vi "ADIS16470 Loop.vi"(8 "error in":errorcluster, 9 "Calibration Time":T5, 11 "ADIS16470DevRef":T7={"DevStatus"={"status"=FALSE, "code"=0, "source"=""}, "Hardware Config"={"SPI Clock Rate (Hz)"=1000000.0, "IMU SPI Mode (3)"=enum."Mode 3 (Clk Idle High,Sample on Trailing)", "IMU Reset Pin"=enum."SPI Port CS2", "IMU SPI Bus"=enum."SPI On-Board, CS0", "IMU Data Ready Pin"=enum."SPI Port CS1", "Stall Config"={"Pow2BytesPerRead"=255, "StallTicks"=640, "CsToSclkTicks"=5}}, "Calibration Complete"=refnum, "Status FIFO"=refnum, "Last Value Reference"=refnum, "Sychronous Process VI"=refnum, "Cmd FIFO"=refnum, "Source"={"DevStatus"={"status"=FALSE, "code"=0, "source"=""}, "AnalogTriggerMode?"=FALSE, "DigitalMode"={"DIO Channel"=enum."Disabled"}, "AnalogTriggerMode"={"AnalogTriggerIndex"=enum."Trig 0", "OutputType"=enum."InWindow"}}, "Data FIFO"=refnum, "Calibration Time"=enum."1s"}) -> ()   [LabVIEW 2019]
uses:
  Typedef/ADIS16470 Device Reference.ctl
  Typedef/ADIS16470 Hardware Configuration.ctl
  <vilib>/Rock Robotics/WPI/SPI/WPI_SPIMode.ctl
  <vilib>/Rock Robotics/SystemInterfaces/DIO/FPGA_DIOChannel.ctl
  <vilib>/Rock Robotics/SystemInterfaces/spilib/spi_bus.ctl
  Typedef/ADIS16470 Status.ctl
  Typedef/ADIS16470 Data.ctl
  Typedef/ADIS16470 Process.ctl
  Typedef/ADIS16470 Command Type.ctl
  <vilib>/Rock Robotics/SystemInterfaces/CounterEncoderSourceConvertion/FPGA_CounterEncoderSourceConvertionLVSourceType.ctl
  <vilib>/Rock Robotics/SystemInterfaces/DIO/FPGA_DIODigitalSourceChannel.ctl
  <vilib>/Rock Robotics/SystemInterfaces/AnalogTrigger/FPGA_AnalogTriggerIndex.ctl
  <vilib>/Rock Robotics/SystemInterfaces/AnalogTrigger/FPGA_AnalogTriggerOutType.ctl
  Typedef/ADIS16470 Calibration Time.ctl
  <vilib>/Rock Robotics/WPI/Encoder/WPI_EncoderDevRef.ctl
  <vilib>/Rock Robotics/SystemInterfaces/Encoder/FPGA_EncoderIdx.ctl
  <vilib>/Rock Robotics/SystemInterfaces/Counter/FPGA_CounterCtrSystemIndex.ctl
  <vilib>/Rock Robotics/WPI/Encoder/WPI_EncoderType.ctl
  <vilib>/Rock Robotics/WPI/SPI/WPI_SPIDevRef.ctl
  Typedef/ADIS16470 Register.ctl
  <vilib>/Rock Robotics/WPI/DMA/WPI_DMARef.ctl
  Typedef/ADIS16470 State Machine.ctl
  <vilib>/Rock Robotics/WPI/DMA/WPI_DMAEncoderOutputType.ctl
  <vilib>/Rock Robotics/WPI/Counter/WPI_CounterDigitalInputToDigitalSource.vi
  <vilib>/Rock Robotics/WPI/DMA/WPI_DMAOpenExternal.vi
  <vilib>/Rock Robotics/WPI/DMA/WPI_DMAAddChannelToStream_Encoder.vi
  <vilib>/Rock Robotics/WPI/DMA/WPI_DMAAddChannelToStream_Timestamp.vi
panel:
  in  "Encoder R":T1={"DevStatus"={"status"=FALSE, "code"=0, "source"=""}, "EncoderIndex"=enum."Invalid", "CounterIndex"=enum."Invalid", "DistancePerCount"=1.0, "Decoding Type"=enum."4x"}
  in  "Encoder L":T1={"DevStatus"={"status"=FALSE, "code"=0, "source"=""}, "EncoderIndex"=enum."Invalid", "CounterIndex"=enum."Invalid", "DistancePerCount"=1.0, "Decoding Type"=enum."4x"}
  in  "element":T6
  out "Waveform Chart":dbl(graph)
  out "Offset Bias":i16[](array[numeric])
  # "XG_BIAS_LOW"
  # "XG_BIAS_HIGH"
  # "YG_BIAS_LOW"
  # "YG_BIAS_HIGH"
  # "ZG_BIAS_LOW"
  # "ZG_BIAS_HIGH"
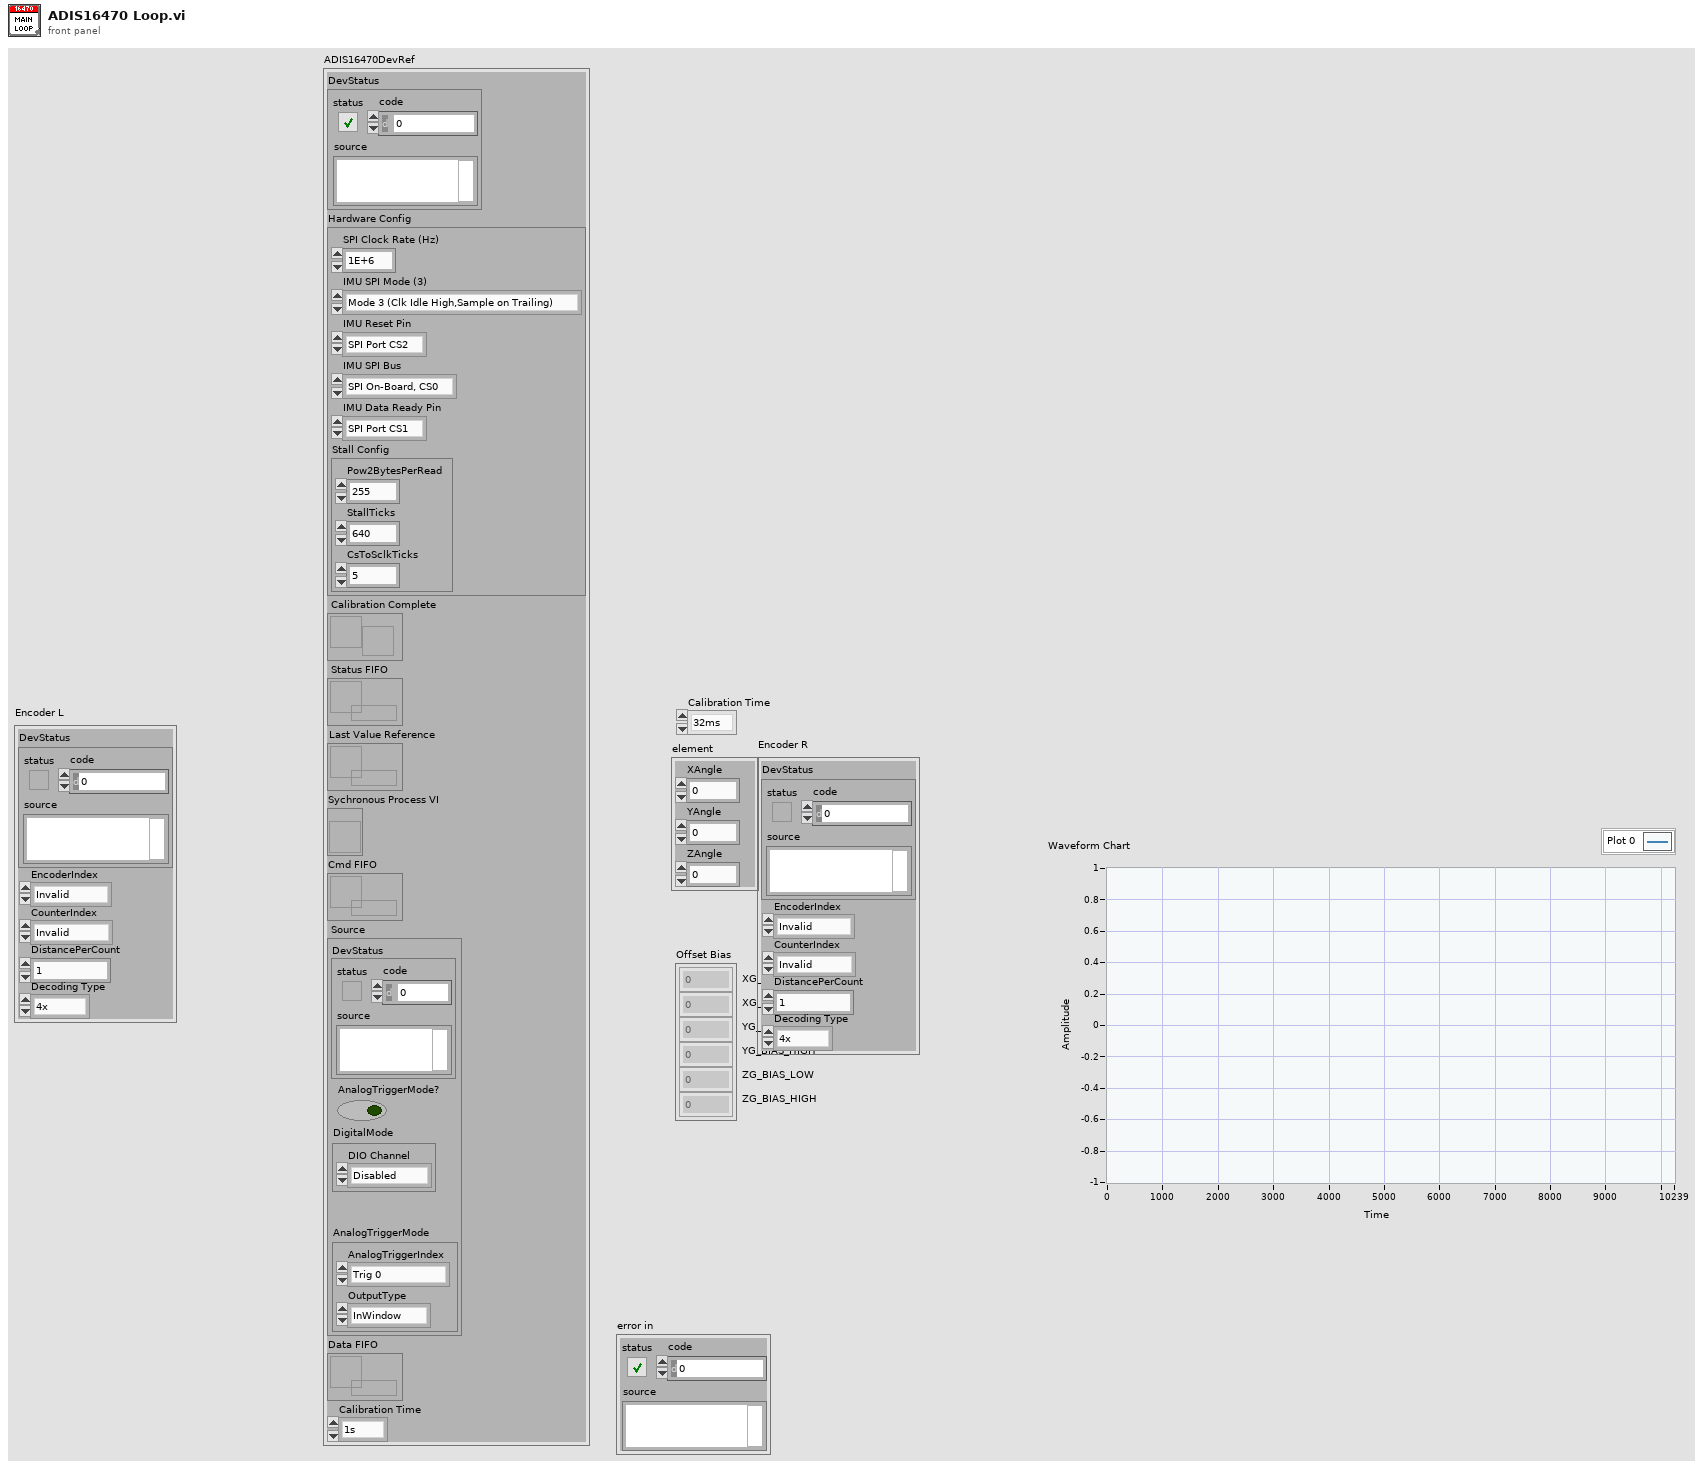
[diagram p1: front panel]
types:
  T1 = typedef "WPI_EncoderDevRef.ctl" = cluster{"DevStatus":errorcluster, "EncoderIndex":T2, "CounterIndex":T3, "DistancePerCount":dbl, "Decoding Type":T4}
  T2 = typedef "FPGA_EncoderIdx.ctl" = enum8{"Enc 0", "Enc 1", "Enc 2", "Enc 3", "Enc 4", "Enc 5", "Enc 6", "Enc 7", "Invalid"}
  T3 = typedef "FPGA_CounterCtrSystemIndex.ctl" = enum8{"Ctr 0", "Ctr 1", "Ctr 2", "Ctr 3", "Ctr 4", "Ctr 5", "Ctr 6", "Ctr 7", "Invalid"}
  T4 = typedef "WPI_EncoderType.ctl" = enum16{"1x", "2x", "4x"}
  T5 = typedef "ADIS16470 Calibration Time.ctl" = enum16{"32ms", "64ms", "128ms", "256ms", "512ms", "1s", "2s", "4s", "8s", "16s", "32s", "64s"}
  T6 = typedef "ADIS16470 Data.ctl" = cluster{"XAngle":dbl, "YAngle":dbl, "ZAngle":dbl}
  T7 = typedef "ADIS16470 Device Reference.ctl" = cluster{"DevStatus":errorcluster, "Hardware Config":T8, "Calibration Complete":refnum<notifier>, "Status FIFO":refnum<k33>, "Last Value Reference":refnum<data-value>, "Sychronous Process VI":T12, "Cmd FIFO":refnum<k33>, "Source":T13, "Data FIFO":refnum<k33>, "Calibration Time":T5}
  T8 = typedef "ADIS16470 Hardware Configuration.ctl" = cluster{"SPI Clock Rate (Hz)":dbl, "IMU SPI Mode (3)":T9, "IMU Reset Pin":T10, "IMU SPI Bus":T11, "IMU Data Ready Pin":T10, "Stall Config":cluster{"Pow2BytesPerRead":u8, "StallTicks":u16, "CsToSclkTicks":u8}}
  T9 = typedef "WPI_SPIMode.ctl" = enum16{"Mode 0 (Clk Idle Low,Sample on Leading)", "Mode 1 (Clk Idle Low,Sample on Trailing)", "Mode 2 (Clk Idle High,Sample on Leading)", "Mode 3 (Clk Idle High,Sample on Trailing)"}
  T10 = typedef "FPGA_DIOChannel.ctl" = enum8{"DIO 0", "DIO 1", "DIO 2", "DIO 3", "DIO 4", "DIO 5", "DIO 6", "DIO 7", "DIO 8", "DIO 9", "DIO MXP 0", "DIO MXP 1", "DIO MXP 2", "DIO MXP 3", "DIO MXP 4", "DIO MXP 5", "DIO MXP 6", "DIO MXP 7", "DIO MXP 8", "DIO MXP 9", "DIO MXP 10", "DIO MXP 11", "DIO MXP 12", "DIO MXP 13", "DIO MXP 14", "DIO MXP 15", "SPI Port CS1", "SPI Port CS2", "SPI Port CS3", "SPI Port MISO", "SPI Port MOSI", "Invalid"}
  T11 = typedef "spi_bus.ctl" = enum16{"SPI On-Board, CS0", "SPI On-Board, CS1", "SPI On-Board, CS2", "SPI On-Board, CS3", "SPI MXP", "Invalid"}
  T12 = typedef "ADIS16470 Process.ctl" = refnum<vi>
  T13 = typedef "FPGA_CounterEncoderSourceConvertionLVSourceType.ctl" = cluster{"DevStatus":errorcluster, "AnalogTriggerMode?":bool, "DigitalMode":cluster{"DIO Channel":T14}, "AnalogTriggerMode":cluster{"AnalogTriggerIndex":T15, "OutputType":T16}}
  T14 = typedef "FPGA_DIODigitalSourceChannel.ctl" = enum8{"DIO 0", "DIO 1", "DIO 2", "DIO 3", "DIO 4", "DIO 5", "DIO 6", "DIO 7", "DIO 8", "DIO 9", "DIO MXP 0", "DIO MXP 1", "DIO MXP 2", "DIO MXP 3", "DIO MXP 4", "DIO MXP 5", "DIO MXP 6", "DIO MXP 7", "DIO MXP 8", "DIO MXP 9", "DIO MXP 10", "DIO MXP 11", "DIO MXP 12", "DIO MXP 13", "DIO MXP 14", "DIO MXP 15", "SPI Port CS1", "SPI Port CS2", "SPI Port CS3", "SPI Port MISO", "SPI Port MOSI", "Disabled"}
  T15 = typedef "FPGA_AnalogTriggerIndex.ctl" = enum8{"Trig 0", "Trig 1", "Trig 2", "Trig 3", "Trig 4", "Trig 5", "Trig 6", "Trig 7", "Invalid"}
  T16 = typedef "FPGA_AnalogTriggerOutType.ctl" = enum16{"InWindow", "TriggerState", "Rising", "Falling"}
  T17 = typedef "ADIS16470 State Machine.ctl" = enum16{"Error", "Reset", "Register DR Source", "Start SPI", "Write Config", "Calibrate", "Write Run Config", "Init Encoder DMA", "Init Auto SPI", "Decode AutoSPI", "Decode Encoder DMA", "Process", "Run Cmds", "Close"}
  T18 = typedef "WPI_SPIDevRef.ctl" = cluster{"DevStatus":errorcluster, "Handle":i32, "SPI Bus":T11}
  T19 = typedef "ADIS16470 Register.ctl" = u8
  T20 = typedef "WPI_DMARef.ctl" = cluster{"DevStatus":errorcluster, "Host Buffer Depth (Samples)":u32}
  T21 = cluster{"SPIDevRef":T18, "Data Counter":u16, "Reset":bool, "Data Ready Source":T13, "Bytes Per Sample":u32, "Data":dbl[], "ADIS16470DevRef":T7, "TimeStampPrev":u32, "Sensor to Robot Rotation":dbl[][], "Data Packet":T19[], "AutoSPI Active?":bool, "Encoder L":T1, "Encoder R":T1, "DMARef":T20}
  T22 = typedef "ADIS16470 Status.ctl" = cluster{"Calibrated?":bool, "IMU Detected?":bool}
  T23 = cluster{"DigitalSource":T13, "Edge":enum16{"Rising Edge", "Falling Edge", "Raising & Falling Edge", "Disabled"}}
  T24 = typedef "ADIS16470 Command Type.ctl" = cluster{"Command":enum16{"None", "Reset", "Set Calibration Period", "Recalibrate", "Recal Complete", "Exit Auto SPI", "Start Auto SPI"}, "Data":u32}
  T25 = typedef "WPI_DigitalOutputDevRef.ctl" = cluster{"DIO Channel":T10, "DevStatus":errorcluster}
  T26 = typedef "WPI_DigitalInputDevRef.ctl" = cluster{"DevStatus":errorcluster, "DIO Channel":T10}
  T27 = typedef "WPI_DMAEncoderOutputType.ctl" = enum16{"Encoder Value", "Timer Value"}
  T28 = cluster{"DigitalSource":T13, "Edge":enum16{"Rising Edge", "Falling Edge", "Raising & Falling Edge", "Disabled"}}[]
  T29 = cluster{"Pow2BytesPerRead":u8, "StallTicks":u16, "CsToSclkTicks":u8}
  T30 = enum16{"None", "Reset", "Set Calibration Period", "Recalibrate", "Recal Complete", "Exit Auto SPI", "Start Auto SPI"}
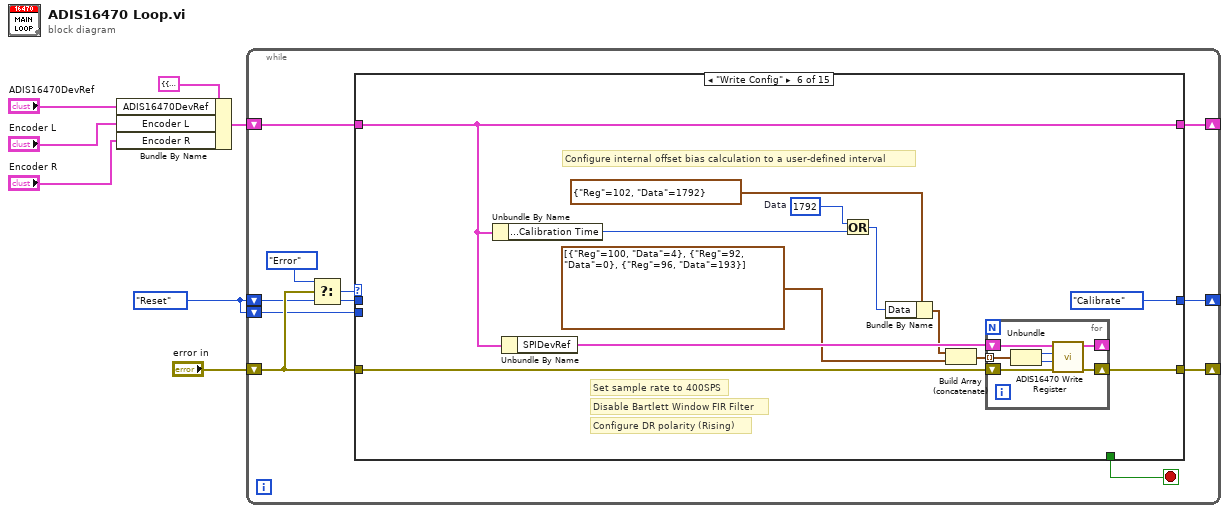
[diagram p0: block diagram]
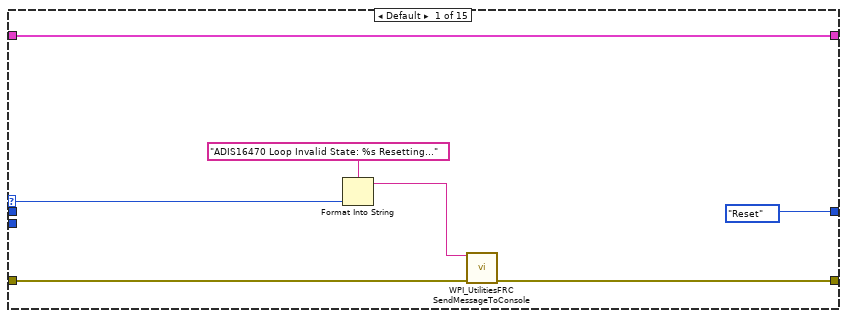
[diagram p2: hidden frame]
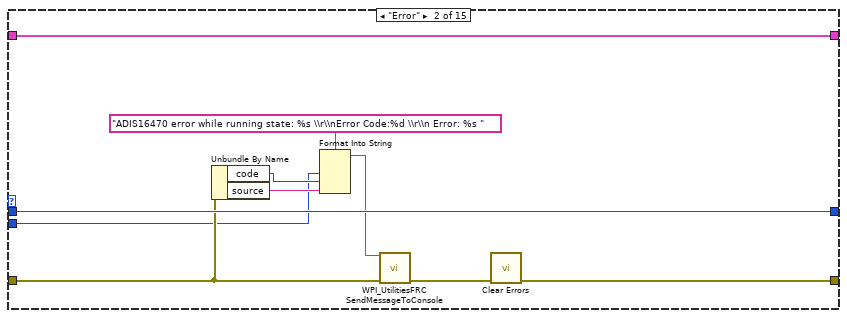
[diagram p3: hidden frame]
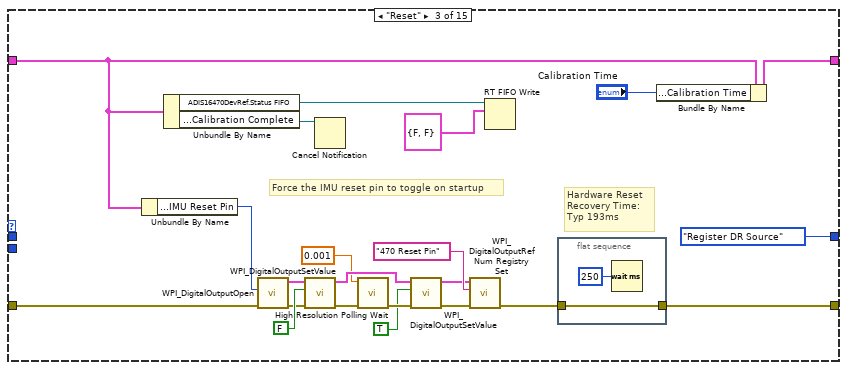
[diagram p4: hidden frame]
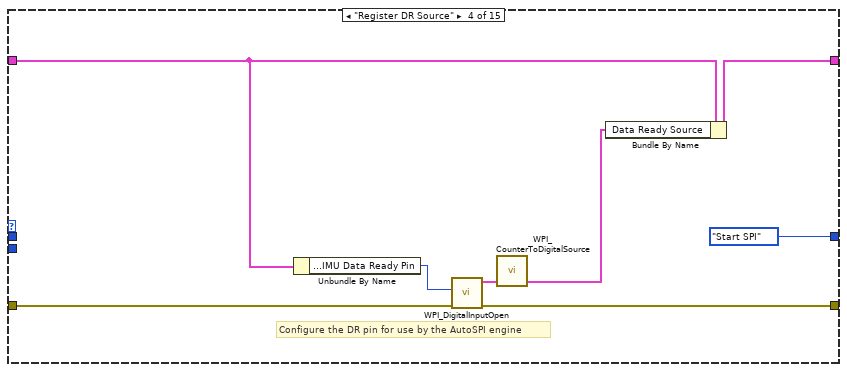
[diagram p5: hidden frame]
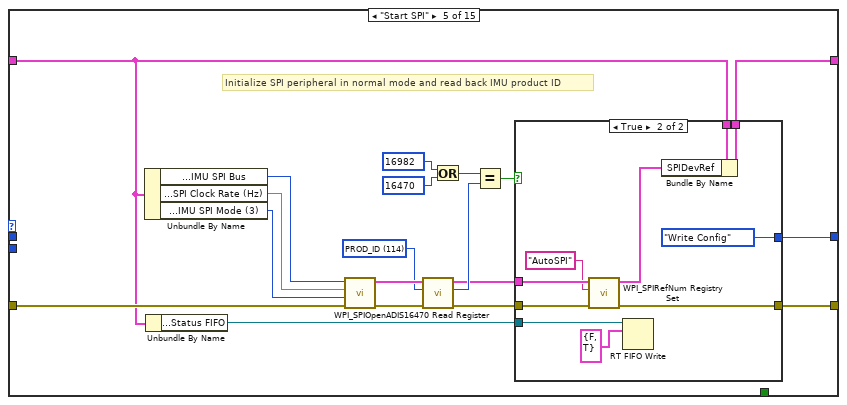
[diagram p6: hidden frame]
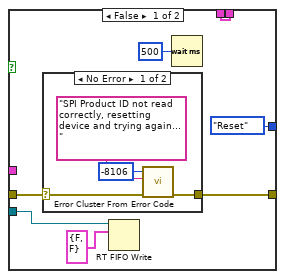
[diagram p7: hidden frame]
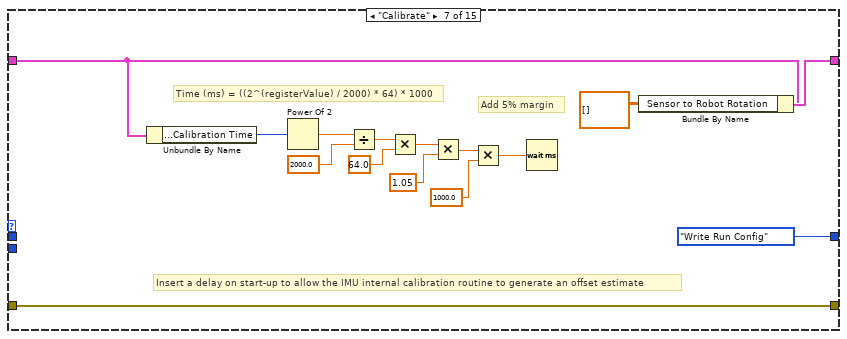
[diagram p9: hidden frame]
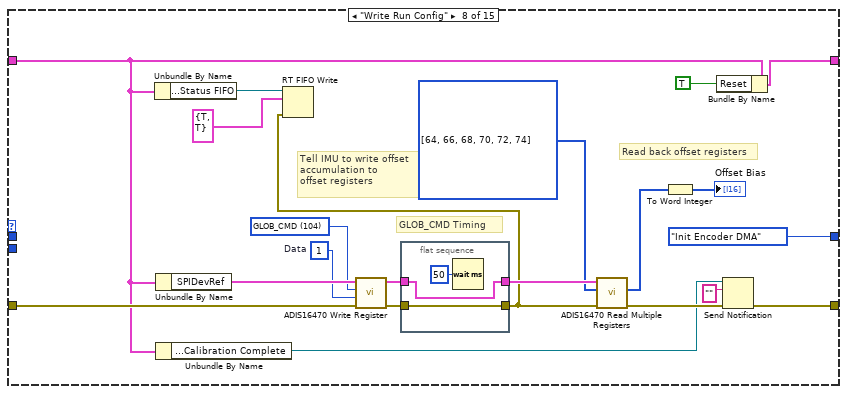
[diagram p10: hidden frame]
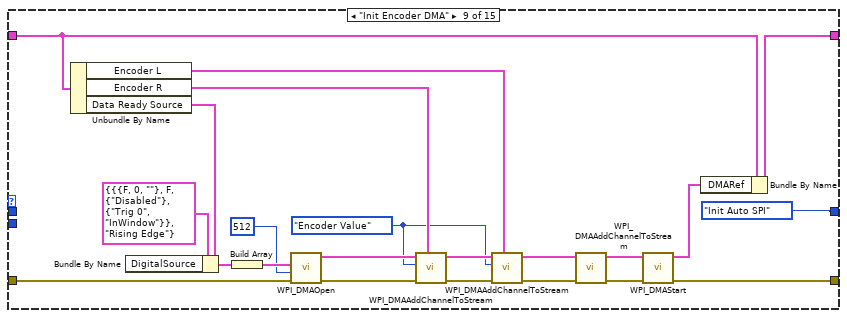
[diagram p11: hidden frame]
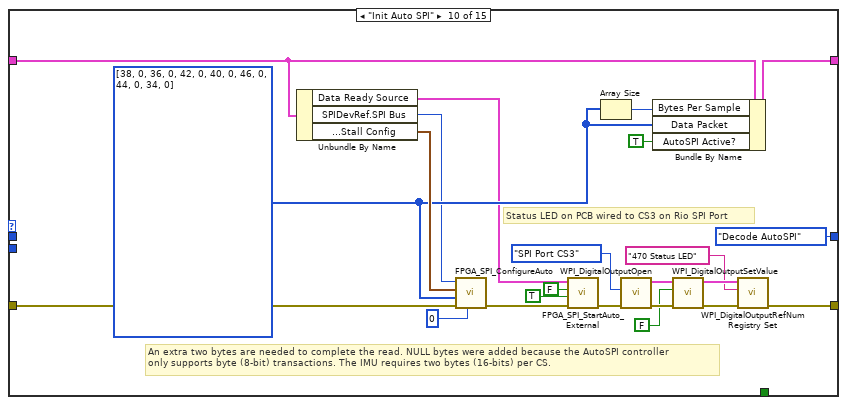
[diagram p12: hidden frame]
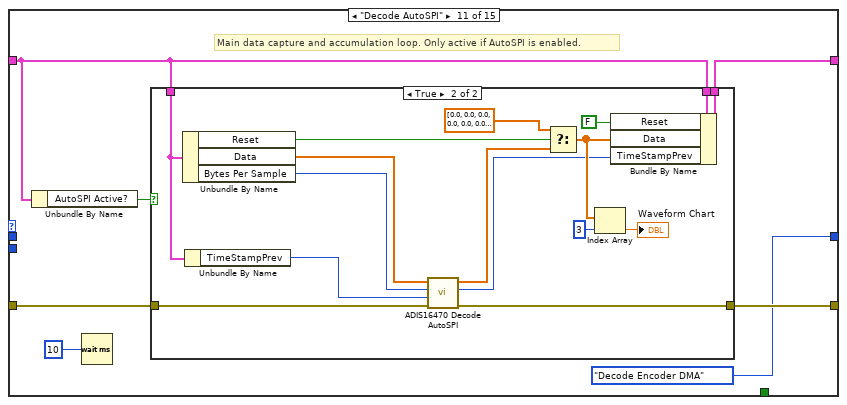
[diagram p13: hidden frame]
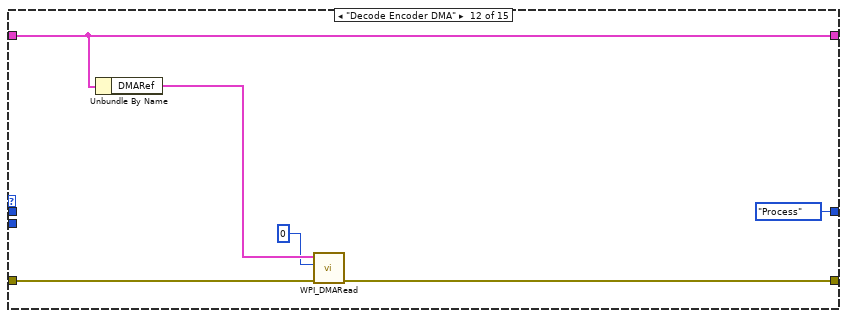
[diagram p15: hidden frame]
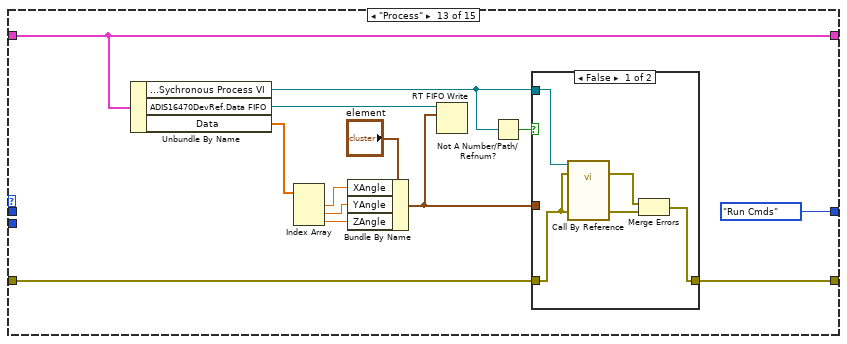
[diagram p16: hidden frame]
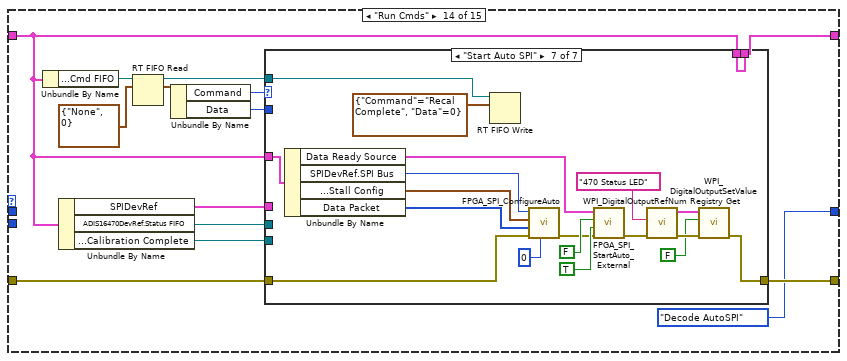
[diagram p18: hidden frame]
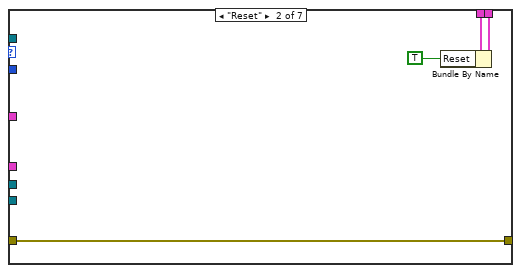
[diagram p20: hidden frame]
diagram:
  w3 = ADIS16470_State_Machine."Reset" ("ADIS16470 State Machine")
  n1 = Bundle By Name(cluster=T21 {"SPIDevRef"={"DevStatus"={"status"=FALSE, "code"=0, "source"=""}, "Handle"=0, "SPI Bus"=enum."SPI On-Board, CS0"}, "Data Counter"=0, "Reset"=FALSE, "Data Ready Source"={"DevStatus"={"status"=FALSE, "code"=0, "source"=""}, "AnalogTriggerMode?"=FALSE, "DigitalMode"={"DIO Channel"=enum."DIO 1"}, "AnalogTriggerMode"={"AnalogTriggerIndex"=enum."Trig 0", "OutputType"=enum."InWindow"}}, "Bytes Per Sample"=0, "Data"=[0.0, 0.0, 0.0, 0.0, 0.0, 0.0, 0.0, 0.0], "ADIS16470DevRef"={"DevStatus"={"status"=FALSE, "code"=0, "source"=""}, "Hardware Config"={"SPI Clock Rate (Hz)"=1000000.0, "IMU SPI Mode (3)"=enum."Mode 3 (Clk Idle High,Sample on Trailing)", "IMU Reset Pin"=enum."SPI Port CS2", "IMU SPI Bus"=enum."SPI On-Board, CS0", "IMU Data Ready Pin"=enum."SPI Port CS1", "Stall Config"={"Pow2BytesPerRead"=255, "StallTicks"=640, "CsToSclkTicks"=5}}, "Calibration Complete"=refnum, "Status FIFO"=refnum, "Last Value Reference"=refnum, "Sychronous Process VI"=refnum, "Cmd FIFO"=refnum, "Source"={"DevStatus"={"status"=FALSE, "code"=0, "source"=""}, "AnalogTriggerMode?"=FALSE, "DigitalMode"={"DIO Channel"=enum."Disabled"}, "AnalogTriggerMode"={"AnalogTriggerIndex"=enum."Trig 0", "OutputType"=enum."InWindow"}}, "Data FIFO"=refnum, "Calibration Time"=enum."1s"}, "TimeStampPrev"=0, "Sensor to Robot Rotation"=[], "Data Packet"=[38, 0, 36, 0, 42, 0, 40, 0, 46, 0, 44, 0, 114, 0], "AutoSPI Active?"=TRUE, "Encoder L"={"DevStatus"={"status"=FALSE, "code"=0, "source"=""}, "EncoderIndex"=enum."Invalid", "CounterIndex"=enum."Invalid", "DistancePerCount"=1.0, "Decoding Type"=enum."4x"}, "Encoder R"={"DevStatus"={"status"=FALSE, "code"=0, "source"=""}, "EncoderIndex"=enum."Invalid", "CounterIndex"=enum."Invalid", "DistancePerCount"=1.0, "Decoding Type"=enum."4x"}, "DMARef"={"DevStatus"={"status"=FALSE, "code"=0, "source"=""}, "Host Buffer Depth (Samples)"=0}}, "ADIS16470DevRef"="ADIS16470DevRef", "Encoder L"="Encoder L", "Encoder R"="Encoder R") -> (w6:T21)
  n2 = while {
    shift-right: [w14] -> _
    shift-left: w3 -> [w11]
    shift-right: [w16] -> _
    shift-left: w6 -> [w17]
    shift-right: [w15] -> _
    shift-left: "error in" -> [w13]
    shift-left: w3 -> [w10]
    stop <- w9 stop-if-true
    n3 = Select(t=ADIS16470_State_Machine."Error" ("ADIS16470 State Machine"), s=w13, f=w11) -> (s? t:f=w12:T17)
    n4 = case shown="\"Write Config\"" w12 {
      selector: w12 -> [w23 _ _ _ _ _ _ _ _ _ _ _ _ _ _]
      tunnel: w17 -> [w24 w34 w38 w63 w68 w110 w138 w148 w187 w203 w213 w240 w254 w263 w389]
      tunnel: [w24 w34 w37 w66 w76 w110 w140 w155 w173 w202 w217 w240 w254 w270 w389] -> w16
      tunnel: w13 -> [w22 w30 w54 w65 w82 w118 w139 w161 w180 w210 w216 w238 w252 w272 w388]
      tunnel: [w21 w31 w53 w60 w75 w117 w139 w150 w168 w194 w215 w237 w251 w271 w388] -> w15
      tunnel: [ADIS16470_State_Machine."Reset" ("ADIS16470 State Machine") w33 ADIS16470_State_Machine."Register DR Source" ("ADIS16470 State Machine") ADIS16470_State_Machine."Start SPI" ("ADIS16470 State Machine") w77 ADIS16470_State_Machine."Calibrate" ("ADIS16470 State Machine") ADIS16470_State_Machine."Write Run Config" ("ADIS16470 State Machine") ADIS16470_State_Machine."Init Encoder DMA" ("ADIS16470 State Machine") ADIS16470_State_Machine."Init Auto SPI" ("ADIS16470 State Machine") ADIS16470_State_Machine."Decode AutoSPI" ("ADIS16470 State Machine") ADIS16470_State_Machine."Decode Encoder DMA" ("ADIS16470 State Machine") ADIS16470_State_Machine."Process" ("ADIS16470 State Machine") ADIS16470_State_Machine."Run Cmds" ("ADIS16470 State Machine") ADIS16470_State_Machine."Decode AutoSPI" ("ADIS16470 State Machine") ADIS16470_State_Machine."Reset" ("ADIS16470 State Machine")] -> w14
      tunnel: w11 -> [_ w33 _ _ _ _ _ _ _ _ _ _ _ _ _]
      tunnel: w10 -> [_ w25 _ _ _ _ _ _ _ _ _ _ _ _ _]
      tunnel: [_ _ _ _ _ _ _ _ _ _ _ _ _ _ TRUE] -> w9
      frame Default {
        n5 = Format Into String(format string="ADIS16470 Loop Invalid State: %s Resetting...", w23) -> (resulting string=w20:string)  [unwired: 2 in, 1 out]
        n6 = call <vilib>:"WPI_UtilitiesFRC SendMessageToConsole.vi"("Message"=w20, "error in (no error)"=w22) -> ("error out"=w21:errorcluster)  [unwired: 13 in]
      }
      frame "Error" {
        n7 = Unbundle By Name(w30) -> ("code"=w27:i32, "source"=w26:string)
        n8 = Format Into String(format string="ADIS16470 error while running state: %s \\r\\nError Code:%d \\r\\n Error: %s ", w25, w27, w26) -> (resulting string=w29:string)  [unwired: 2 in, 1 out]
        n9 = call <vilib>:"WPI_UtilitiesFRC SendMessageToConsole.vi"("Message"=w29, "error in (no error)"=w30) -> ("error out"=w32:errorcluster)  [unwired: 13 in]
        n10 = call <vilib>:"Clear Errors.vi"("error in (no error)"=w32) -> ("error out"=w31:errorcluster)  [unwired: 5 in, 1 out]
      }
      frame "Reset" {
        # "Hardware Reset Recovery Time: Typ 193ms"
        # "Force the IMU reset pin to toggle on startup"
        n11 = Unbundle By Name(w38) -> ("ADIS16470DevRef.Hardware Config.IMU Reset Pin"=w55:T10)
        n12 = Unbundle By Name(w38) -> ("ADIS16470DevRef.Status FIFO"=w51:refnum<k33>, "ADIS16470DevRef.Calibration Complete"=w52:refnum<notifier>)
        n13 = call <vilib>:"WPI_DigitalOutputOpen.vi"("error in (no error)"=w54, "DIO Channel"=w55) -> ("error out"=w48:errorcluster, "DigitalOutputDevRef"=w56:T25)  [unwired: 8 in]
        n14 = call <vilib>:"WPI_DigitalOutputSetValue.vi"("error in (no error)"=w48, "Value"=FALSE, "DigitalOutputDevRef"=w56) -> ("error out"=w45:errorcluster, "DigitalOutputDevRef"=w43:T25)  [unwired: 7 in]
        n15 = Cancel Notification(0:w52) -> ()  [unwired: 1 in, 3 out]
        n16 = call <vilib>:"High Resolution Polling Wait.vi"("error in (no error)"=w45, "seconds to wait"=0.001) -> ("error out"=w44:errorcluster)  [unwired: 9 in]
        n17 = call <vilib>:"WPI_DigitalOutputSetValue.vi"("error in (no error)"=w44, "Value"=TRUE, "DigitalOutputDevRef"=w43) -> ("error out"=w40:errorcluster, "DigitalOutputDevRef"=w41:T25)  [unwired: 7 in]
        n18 = call <vilib>:"WPI_DigitalOutputRefNum Registry Set.vi"("error in (no error)"=w40, "refnum name"="470 Reset Pin", "DigitalOutputDevRef"=w41) -> ("error out"=w46:errorcluster)  [unwired: 7 in, 1 out]
        n19 = RT FIFO Write(0:w51, 1:T22 {"Calibrated?"=FALSE, "IMU Detected?"=FALSE} ("element")) -> ()  [unwired: 3 in, 4 out]
        n20 = flat-sequence {
          tunnel: [w58] -> w53
          tunnel: w46 -> [w58]
          frame #0 {
            n21 = Wait (ms)(milliseconds to wait=u32 250) -> ()  [unwired: 1 out]
          }
        }
        n22 = Bundle By Name(cluster=w38, "ADIS16470DevRef.Calibration Time"="Calibration Time") -> (w37:T21)
      }
      frame "Register DR Source" {
        # "Configure the DR pin for use by the AutoSPI engine"
        n23 = Unbundle By Name(w63) -> ("ADIS16470DevRef.Hardware Config.IMU Data Ready Pin"=w62:T10)
        n24 = call <vilib>:"WPI_DigitalInputOpen.vi"("error in (no error)"=w65, "DIO Channel"=w62) -> ("error out"=w60:errorcluster, "DigitalInputDevRef"=w64:T26)  [unwired: 8 in]
        n25 = call-poly <vilib>:"WPI_CounterToDigitalSource.vi"("DigitalInputDevRef"=w64) -> ("Digital Source"=w61:T13)  [unwired: 6 in]
        n26 = Bundle By Name(cluster=w63, "Data Ready Source"=w61) -> (w66:T21)
      }
      frame "Start SPI" {
        w70 = T19 114 items=["Reserved1"=0, "DIAG_STAT"=2, "X_GYRO_LOW"=4, "X_GYRO_OUT"=6, "Y_GYRO_LOW"=8, "Y_GYRO_OUT"=10, "Z_GYRO_LOW"=12, "Z_GYRO_OUT"=14, "X_ACCL_LOW"=16, "X_ACCL_OUT"=18, "Y_ACCL_LOW"=20, "Y_ACCL_OUT"=22, "Z_ACCL_LOW"=24, "Z_ACCL_OUT"=26, "TEMP_OUT"=28, "TIME_STAMP"=30, "Reseved2"=32, "DATA_CNTR"=34, "X_DELTANG_LOW"=36, "X_DELTANG_OUT"=38, "Y_DELTANG_LOW"=40, "Y_DELTANG_OUT"=42, "Z_DELTANG_LOW"=44, "Z_DELTANG_OUT"=46, "X_DELTVEL_LOW"=48, "X_DELTVEL_OUT"=50, "Y_DELTVEL_LOW"=52, "Y_DELTVEL_OUT"=54, "Z_DELTVEL_LOW"=56, "Z_DELTVEL_OUT"=58, "Reserved3"=60, "Reserved4"=62, "XG_BIAS_LOW"=64, "XG_BIAS_HIGH"=66, "YG_BIAS_LOW"=68, "YG_BIAS_OUT"=70, "ZG_BIAS_LOW"=72, "ZG_BIAS_OUT"=74, "XA_BIAS_LOW"=76, "XA_BIAS_HIGH"=78, "YA_BIAS_LOW"=80, "YA_BIAS_OUT"=82, "ZA_BIAS_LOW"=84, "ZA_BIAS_OUT"=86, "Reserved5"=88, "Reserved6"=90, "FILT_CTRL"=92, "Reserved5"=94, "MSC_CTRL"=96, "UP_SCALE"=98, "DEC_RATE"=100, "NULL_CNFG"=102, "GLOB_CMD"=104, "Reserved6"=106, "FIRM_REV"=108, "FIRM_DM"=110, "FIRM_Y"=112, "PROD_ID"=114, "SERIAL_NUM"=116, "USER_SCR1"=118, "USER_SCR2"=120, "USER_SCR3"=122, "FLSHCNT_LOW"=124, "FLSHCNT_HIGH"=126] ("ADIS16448 Register")
        # "Initialize SPI peripheral in normal mode and read back IMU product ID"
        n27 = Unbundle By Name(w68) -> ("ADIS16470DevRef.Hardware Config.IMU SPI Bus"=w78:T11, "ADIS16470DevRef.Hardware Config.SPI Clock Rate (Hz)"=w79:dbl, "ADIS16470DevRef.Hardware Config.IMU SPI Mode (3)"=w80:T9)
        n28 = Unbundle By Name(w68) -> ("ADIS16470DevRef.Status FIFO"=w67:refnum<k33>)
        n29 = call <vilib>:"WPI_SPIOpen.vi"("error in"=w82, "Mode (3)"=w80, "Clock Rate (Hz)"=w79, "SPI Bus"=w78) -> ("error out"=w72:errorcluster, "SPIDevRef"=w71:T18)  [unwired: 6 in]
        n30 = call "ADIS16470 Read Register.vi"("error in (no error)"=w72, "ADIS16470 Register"=w70, "SPIDevRef in"=w71) -> ("error out"=w73:errorcluster, "Register Value"=w74:u16, "SPIDevRef out"=w69:T18)  [unwired: 6 in]
        n31 = Or(x=u16 16982 ("y"), y=u16 16470) -> (x .or. y?=w83:u16)
        n32 = Equal?(x=w83, y=w74) -> (x = y?=w81:bool)
        n33 = case shown="True" w81 {
          tunnel: [ADIS16470_State_Machine."Reset" ("ADIS16470 State Machine") ADIS16470_State_Machine."Write Config" ("ADIS16470 State Machine")] -> w77
          tunnel: w68 -> [w92 w107]
          tunnel: [w92 w106] -> w76
          tunnel: [w91 w102] -> w75
          tunnel: w73 -> [w90 w105]
          tunnel: w69 -> [_ w104]
          tunnel: w67 -> [w88 w100]
          frame False {
            n34 = case shown="No Error" w90 {
              selector: w90 -> [w95 w97]
              tunnel: [w96 w97] -> w91
              frame No Error {
                n35 = call <vilib>:"Error Cluster From Error Code.vi"("error in (no error)"=w95, "error message (\"\")"="SPI Product ID not read correctly, resetting device and trying again..." ("error message (\"\")"), "error code (0)"=-8106) -> ("error out"=w96:errorcluster)  [unwired: 6 in]
              }
              frame Error {
              }
            }
            n36 = RT FIFO Write(0:w88, 1:T22 {"Calibrated?"=FALSE, "IMU Detected?"=FALSE} ("element")) -> ()  [unwired: 3 in, 4 out]
            n37 = Wait (ms)(milliseconds to wait=u32 500) -> ()  [unwired: 1 out]
          }
          frame True {
            n38 = call <vilib>:"WPI_SPIRefNum Registry Set.vi"("error in (no error)"=w105, "refnum name"="AutoSPI", "SPIDevRef"=w104) -> ("error out"=w102:errorcluster, "SPIDevRef"=w103:T18)  [unwired: 7 in]
            n39 = RT FIFO Write(0:w100, 1:T22 {"Calibrated?"=FALSE, "IMU Detected?"=TRUE} ("element")) -> ()  [unwired: 3 in, 4 out]
            n40 = Bundle By Name(cluster=w107, "SPIDevRef"=w103) -> (w106:T21)
          }
        }
      }
      frame "Write Config" {
        w112 = 1792  # Data
        # "Set sample rate to 400SPS"
        # "Configure internal offset bias calculation to a user-defined interval"
        # "Configure DR polarity (Rising)"
        # "Disable Bartlett Window FIR Filter"
        n41 = Unbundle By Name(w110) -> ("ADIS16470DevRef.Calibration Time"=w109:T5)
        n42 = Unbundle By Name(w110) -> ("SPIDevRef"=w119:T18)
        n43 = Or(x=w112, y=w109) -> (x .or. y?=w111:i32)
        n44 = Bundle By Name(cluster=cluster{"Reg":T19, "Data":i32} {"Reg"=102, "Data"=1792}, "Data"=w111) -> (w113:cluster{"Reg":T19, "Data":i32})
        n45 = Build Array (concatenate)(w113, cluster{"Reg":T19, "Data":u16}[] [{"Reg"=100, "Data"=4}, {"Reg"=92, "Data"=0}, {"Reg"=96, "Data"=193}]) -> (w114:cluster{"Reg":T19, "Data":i32}[])
        n46 = for {
          tunnel: w114 -> [w126] mode=indexing
          shift-right: [w122] -> w117
          shift-left: w118 -> [w121]
          shift-right: [w120] -> _
          shift-left: w119 -> [w123]
          n47 = Unbundle(w126) -> ("Reg"=w125:T19, "Data"=w124:i32)
          n48 = call "ADIS16470 Write Register.vi"("error in (no error)"=w121, "Data"=w124, "Register"=w125, "SPIDevRef in"=w123) -> ("error out"=w122:errorcluster, "SPIDevRef out"=w120:T18)  [unwired: 6 in]
        }
      }
      frame "Calibrate" {
        # "Insert a delay on start-up to allow the IMU internal calibration routine to generate an offset estimate"
        # "Add 5% margin"
        # "Time (ms) = ((2^(registerValue) / 2000) * 64) * 1000"
        n49 = Unbundle By Name(w138) -> ("ADIS16470DevRef.Calibration Time"=w137:T5)
        n50 = Power Of 2(x=w137) -> (2^x=w136:dbl)
        n51 = Divide(x=w136, y=2000.0) -> (x/y=w134:dbl)
        n52 = Multiply(x=w134, y=64.0) -> (x*y=w132:dbl)
        n53 = Multiply(x=w132, y=1.05) -> (x*y=w130:dbl)
        n54 = Multiply(x=w130, y=1000.0) -> (x*y=w128:dbl)
        n55 = Wait (ms)(milliseconds to wait=w128) -> ()  [unwired: 1 out]
        n56 = Bundle By Name(cluster=w138, "Sensor to Robot Rotation"=dbl[][] []) -> (w140:T21)
      }
      frame "Write Run Config" {
        w145 = T19 104 items=["Reserved1"=0, "DIAG_STAT"=2, "X_GYRO_LOW"=4, "X_GYRO_OUT"=6, "Y_GYRO_LOW"=8, "Y_GYRO_OUT"=10, "Z_GYRO_LOW"=12, "Z_GYRO_OUT"=14, "X_ACCL_LOW"=16, "X_ACCL_OUT"=18, "Y_ACCL_LOW"=20, "Y_ACCL_OUT"=22, "Z_ACCL_LOW"=24, "Z_ACCL_OUT"=26, "TEMP_OUT"=28, "TIME_STAMP"=30, "Reseved2"=32, "DATA_CNTR"=34, "X_DELTANG_LOW"=36, "X_DELTANG_OUT"=38, "Y_DELTANG_LOW"=40, "Y_DELTANG_OUT"=42, "Z_DELTANG_LOW"=44, "Z_DELTANG_OUT"=46, "X_DELTVEL_LOW"=48, "X_DELTVEL_OUT"=50, "Y_DELTVEL_LOW"=52, "Y_DELTVEL_OUT"=54, "Z_DELTVEL_LOW"=56, "Z_DELTVEL_OUT"=58, "Reserved3"=60, "Reserved4"=62, "XG_BIAS_LOW"=64, "XG_BIAS_HIGH"=66, "YG_BIAS_LOW"=68, "YG_BIAS_OUT"=70, "ZG_BIAS_LOW"=72, "ZG_BIAS_OUT"=74, "XA_BIAS_LOW"=76, "XA_BIAS_HIGH"=78, "YA_BIAS_LOW"=80, "YA_BIAS_OUT"=82, "ZA_BIAS_LOW"=84, "ZA_BIAS_OUT"=86, "Reserved5"=88, "Reserved6"=90, "FILT_CTRL"=92, "Reserved5"=94, "MSC_CTRL"=96, "UP_SCALE"=98, "DEC_RATE"=100, "NULL_CNFG"=102, "GLOB_CMD"=104, "Reserved6"=106, "FIRM_REV"=108, "FIRM_DM"=110, "FIRM_Y"=112, "PROD_ID"=114, "SERIAL_NUM"=116, "USER_SCR1"=118, "USER_SCR2"=120, "USER_SCR3"=122, "FLSHCNT_LOW"=124, "FLSHCNT_HIGH"=126] ("Register")
        w160 = u16 1  # Data
        w156 = T19[] [64, 66, 68, 70, 72, 74] items=["Reserved1"=0, "DIAG_STAT"=2, "X_GYRO_LOW"=4, "X_GYRO_OUT"=6, "Y_GYRO_LOW"=8, "Y_GYRO_OUT"=10, "Z_GYRO_LOW"=12, "Z_GYRO_OUT"=14, "X_ACCL_LOW"=16, "X_ACCL_OUT"=18, "Y_ACCL_LOW"=20, "Y_ACCL_OUT"=22, "Z_ACCL_LOW"=24, "Z_ACCL_OUT"=26, "TEMP_OUT"=28, "TIME_STAMP"=30, "Reseved2"=32, "DATA_CNTR"=34, "X_DELTANG_LOW"=36, "X_DELTANG_OUT"=38, "Y_DELTANG_LOW"=40, "Y_DELTANG_OUT"=42, "Z_DELTANG_LOW"=44, "Z_DELTANG_OUT"=46, "X_DELTVEL_LOW"=48, "X_DELTVEL_OUT"=50, "Y_DELTVEL_LOW"=52, "Y_DELTVEL_OUT"=54, "Z_DELTVEL_LOW"=56, "Z_DELTVEL_OUT"=58, "Reserved3"=60, "Reserved4"=62, "XG_BIAS_LOW"=64, "XG_BIAS_HIGH"=66, "YG_BIAS_LOW"=68, "YG_BIAS_HIGH"=70, "ZG_BIAS_LOW"=72, "ZG_BIAS_HIGH"=74, "XA_BIAS_LOW"=76, "XA_BIAS_HIGH"=78, "YA_BIAS_LOW"=80, "YA_BIAS_HIGH"=82, "ZA_BIAS_LOW"=84, "ZA_BIAS_HIGH"=86, "Reserved5"=88, "Reserved6"=90, "FILT_CTRL"=92, "Reserved5"=94, "MSC_CTRL"=96, "UP_SCALE"=98, "DEC_RATE"=100, "NULL_CNFG"=102, "GLOB_CMD"=104, "Reserved6"=106, "FIRM_REV"=108, "FIRM_DM"=110, "FIRM_Y"=112, "PROD_ID"=114, "SERIAL_NUM"=116, "USER_SCR1"=118, "USER_SCR2"=120, "USER_SCR3"=122, "FLSHCNT_LOW"=124, "FLSHCNT_HIGH"=126] ("Registers")
        # "Tell IMU to write offset \naccumulation to \noffset registers"
        # "GLOB_CMD Timing"
        # "Read back offset registers"
        n57 = Unbundle By Name(w148) -> ("ADIS16470DevRef.Status FIFO"=w147:refnum<k33>)
        n58 = Unbundle By Name(w148) -> ("SPIDevRef"=w162:T18)
        n59 = Unbundle By Name(w148) -> ("ADIS16470DevRef.Calibration Complete"=w151:refnum<notifier>)
        n60 = RT FIFO Write(0:w147, 1:T22 {"Calibrated?"=TRUE, "IMU Detected?"=TRUE} ("element"), 3:w144) -> ()  [unwired: 2 in, 4 out]
        n61 = call "ADIS16470 Write Register.vi"("error in (no error)"=w161, "Data"=w160, "Register"=w145, "SPIDevRef in"=w162) -> ("error out"=w159:errorcluster, "SPIDevRef out"=w158:T18)  [unwired: 6 in]
        n62 = flat-sequence {
          tunnel: w159 -> [w165]
          tunnel: [w165] -> w144
          tunnel: w158 -> [w163]
          tunnel: [w163] -> w157
          frame #0 {
            n63 = Wait (ms)(milliseconds to wait=u32 50) -> ()  [unwired: 1 out]
          }
        }
        n64 = call "ADIS16470 Read Multiple Registers.vi"("error in (no error)"=w144, "Registers"=w156, "SPIDevRefIn"=w157) -> ("error out"=w152:errorcluster, "Values"=w143:u16[])  [unwired: 6 in, 1 out]
        n65 = To Word Integer(number=w143) -> (16bit integer=→"Offset Bias":i16[])
        n66 = Bundle By Name(cluster=w148, "Reset"=TRUE ("First Run")) -> (w155:T21)
        n67 = Send Notification(notification="", notifier=w151, error in (no error)=w152) -> (error out=w150:errorcluster)  [unwired: 1 out]
      }
      frame "Init Encoder DMA" {
        w170 = WPI_DMAEncoderOutputType."Encoder Value" ("Encoder Output Type")
        n68 = Unbundle By Name(w187) -> ("Encoder L"=w172:T1, "Encoder R"=w171:T1, "Data Ready Source"=w183:T13)
        n69 = Bundle By Name(cluster=T23 {"DigitalSource"={"DevStatus"={"status"=FALSE, "code"=0, "source"=""}, "AnalogTriggerMode?"=FALSE, "DigitalMode"={"DIO Channel"=enum."Disabled"}, "AnalogTriggerMode"={"AnalogTriggerIndex"=enum."Trig 0", "OutputType"=enum."InWindow"}}, "Edge"=enum."Rising Edge"} ("ExternalSampleClock"), "DigitalSource"=w183) -> (w182:T23)
        n70 = Build Array(w182) -> (w181:T28)
        n71 = call-poly <vilib>:"WPI_DMAOpen.vi"("error in (no error)"=w180, "Host Buffer Depth (Samples)"=u32 512, "ExternalSampleClocks"=w181) -> ("error out"=w179:errorcluster, "DMARef"=w186:T20)  [unwired: 7 in]
        n72 = call-poly <vilib>:"WPI_DMAAddChannelToStream.vi"("EncoderDevRef"=w171, "error in (no error)"=w179, "Encoder Output Type"=w170, "DMARef"=w186) -> ("error out"=w178:errorcluster, "DMARef"=w185:T20)  [unwired: 6 in]
        n73 = call-poly <vilib>:"WPI_DMAAddChannelToStream.vi"("EncoderDevRef"=w172, "error in (no error)"=w178, "Encoder Output Type"=w170, "DMARef"=w185) -> ("error out"=w174:errorcluster, "DMARef"=w176:T20)  [unwired: 6 in]
        n74 = call-poly <vilib>:"WPI_DMAAddChannelToStream.vi"("error in (no error)"=w174, "DMARef"=w176) -> ("error out"=w175:errorcluster, "DMARef"=w167:T20)  [unwired: 8 in]
        n75 = call <vilib>:"WPI_DMAStart.vi"("error in (no error)"=w175, "DMARef"=w167) -> ("error out"=w168:errorcluster, "DMARef"=w166:T20)  [unwired: 8 in]
        n76 = Bundle By Name(cluster=w187, "DMARef"=w166) -> (w173:T21)
      }
      frame "Init Auto SPI" {
        w191 = T19[] [38, 0, 36, 0, 42, 0, 40, 0, 46, 0, 44, 0, 34, 0] items=["NULL"=0, "DIAG_STAT"=2, "X_GYRO_LOW"=4, "X_GYRO_OUT"=6, "Y_GYRO_LOW"=8, "Y_GYRO_OUT"=10, "Z_GYRO_LOW"=12, "Z_GYRO_OUT"=14, "X_ACCL_LOW"=16, "X_ACCL_OUT"=18, "Y_ACCL_LOW"=20, "Y_ACCL_OUT"=22, "Z_ACCL_LOW"=24, "Z_ACCL_OUT"=26, "TEMP_OUT"=28, "TIME_STAMP"=30, "Reseved2"=32, "DATA_CNTR"=34, "X_DELTANG_LOW"=36, "X_DELTANG_OUT"=38, "Y_DELTANG_LOW"=40, "Y_DELTANG_OUT"=42, "Z_DELTANG_LOW"=44, "Z_DELTANG_OUT"=46, "X_DELTVEL_LOW"=48, "X_DELTVEL_OUT"=50, "Y_DELTVEL_LOW"=52, "Y_DELTVEL_OUT"=54, "Z_DELTVEL_LOW"=56, "Z_DELTVEL_OUT"=58, "Reserved3"=60, "Reserved4"=62, "XG_BIAS_LOW"=64, "XG_BIAS_HIGH"=66, "YG_BIAS_LOW"=68, "YG_BIAS_HIGH"=70, "ZG_BIAS_LOW"=72, "ZG_BIAS_HIGH"=74, "XA_BIAS_LOW"=76, "XA_BIAS_HIGH"=78, "YA_BIAS_LOW"=80, "YA_BIAS_HIGH"=82, "ZA_BIAS_LOW"=84, "ZA_BIAS_HIGH"=86, "Reserved5"=88, "Reserved6"=90, "FILT_CTRL"=92, "Reserved5"=94, "MSC_CTRL"=96, "UP_SCALE"=98, "DEC_RATE"=100, "NULL_CNFG"=102, "GLOB_CMD"=104, "Reserved6"=106, "FIRM_REV"=108, "FIRM_DM"=110, "FIRM_Y"=112, "PROD_ID"=114, "SERIAL_NUM"=116, "USER_SCR1"=118, "USER_SCR2"=120, "USER_SCR3"=122, "FLSHCNT_LOW"=124, "FLSHCNT_HIGH"=126] ("Registers")
        # "Status LED on PCB wired to CS3 on Rio SPI Port"
        # "An extra two bytes are needed to complete the read. NULL bytes were added because the AutoSPI controller \nonly supports byte (8-bit) transactions. The IMU requires two bytes (16-bits) per CS."
        n77 = Unbundle By Name(w203) -> ("Data Ready Source"=w190:T13, "SPIDevRef.SPI Bus"=w189:T11, "ADIS16470DevRef.Hardware Config.Stall Config"=w193:T29)
        n78 = call <vilib>:"FPGA_SPI_ConfigureAuto.vi"("SPI Auto Zero Byte Count"=u8 0, "error in"=w210, "SPI Auto TX Byte Array"=w191, "Stall Config"=w193, "SPI Bus"=w189) -> ("error out"=w208:errorcluster)  [unwired: 6 in]
        n79 = call <vilib>:"FPGA_SPI_StartAuto_External.vi"("error in (no error)"=w208, "Falling Edge"=TRUE, "Rising Edge"=FALSE, "Source"=w190) -> ("error out"=w204:errorcluster)  [unwired: 7 in]
        n80 = Array Size(array=w191) -> (size(s)=w201:i32)
        n81 = call <vilib>:"WPI_DigitalOutputOpen.vi"("error in (no error)"=w204, "DIO Channel"=FPGA_DIOChannel."SPI Port CS3") -> ("error out"=w200:errorcluster, "DigitalOutputDevRef"=w199:T25)  [unwired: 8 in]
        n82 = Bundle By Name(cluster=w203, "Bytes Per Sample"=w201, "Data Packet"=w191, "AutoSPI Active?"=TRUE) -> (w202:T21)
        n83 = call <vilib>:"WPI_DigitalOutputSetValue.vi"("error in (no error)"=w200, "Value"=FALSE, "DigitalOutputDevRef"=w199) -> ("error out"=w197:errorcluster, "DigitalOutputDevRef"=w196:T25)  [unwired: 7 in]
        n84 = call <vilib>:"WPI_DigitalOutputRefNum Registry Set.vi"("error in (no error)"=w197, "refnum name"="470 Status LED", "DigitalOutputDevRef"=w196) -> ("error out"=w194:errorcluster)  [unwired: 7 in, 1 out]
      }
      frame "Decode AutoSPI" {
        # "Main data capture and accumulation loop. Only active if AutoSPI is enabled."
        n85 = Unbundle By Name(w213) -> ("AutoSPI Active?"=w212:bool)
        n86 = Wait (ms)(milliseconds to wait=u32 10) -> ()  [unwired: 1 out]
        n87 = case shown="True" w212 {
          tunnel: [w219 w235] -> w217
          tunnel: w216 -> [w218 w223]
          tunnel: [w218 w221] -> w215
          tunnel: w213 -> [w219 w226]
          tunnel: w213 -> [_ w224]
          frame False {
          }
          frame True {
            n88 = Unbundle By Name(w224) -> ("Reset"=w233:bool, "Data"=w231:dbl[], "Bytes Per Sample"=w232:u32)
            n89 = Unbundle By Name(w224) -> ("TimeStampPrev"=w222:u32)
            n90 = call "ADIS16470 Decode AutoSPI.vi"("error in (no error)"=w223, "TimeStampPrev"=w222, "Bytes Per Sample"=w232, "Data in"=w231) -> ("error out"=w221:errorcluster, "Last Timestamp"=w225:u32, "Data out"=w230:dbl[])  [unwired: 5 in]
            n91 = Select(t=dbl[] [0.0, 0.0, 0.0, 0.0, 0.0, 0.0, 0.0, 0.0] ("Angle and Vel"), s=w233, f=w230) -> (s? t:f=w229:dbl[])
            n92 = Index Array(array=w229, index=3) -> (element=→"Waveform Chart":dbl)
            n93 = Bundle By Name(cluster=w226, "Reset"=FALSE ("First Run"), "Data"=w229, "TimeStampPrev"=w225) -> (w235:T21)
          }
        }
      }
      frame "Decode Encoder DMA" {
        n94 = Unbundle By Name(w240) -> ("DMARef"=w239:T20)
        n95 = call <vilib>:"WPI_DMARead.vi"("error in (no error)"=w238, "SamplesToRead"=u32 0, "DMARef"=w239) -> ("error out"=w237:errorcluster)  [unwired: 3 in, 5 out]
      }
      frame "Process" {
        n96 = Unbundle By Name(w254) -> ("ADIS16470DevRef.Sychronous Process VI"=w249:T12, "ADIS16470DevRef.Data FIFO"=w253:refnum<k33>, "Data"=w248:dbl[])
        n97 = Index Array(array=w248) -> (element #1=w247:dbl, element #2=w246:dbl, element #3=w245:dbl)  [unwired: 3 in]
        n98 = Bundle By Name(cluster="element", "XAngle"=w247, "YAngle"=w246, "ZAngle"=w245) -> (w243:T6)
        n99 = RT FIFO Write(0:w253, 1:w243) -> ()  [unwired: 3 in, 4 out]
        n100 = Not A Number/Path/Refnum?(number/path/refnum=w249) -> (NaN/Path/Refnum?=w250:bool)
        n101 = case shown="False" w250 {
          tunnel: w252 -> [w255 w260]
          tunnel: w243 -> [_ _]
          tunnel: [w259 w260] -> w251
          tunnel: w249 -> [w258 _]
          frame False {
            n102 = call-by-ref "?"(reference=w258, error in=w255, 8:"error in (no error)"=w255) -> (error out=w256:errorcluster, 0:"error out"=w257:errorcluster)  [unwired: 10 in, 1 out]
            n103 = Merge Errors(w256, w257) -> (w259:errorcluster)
          }
          frame True {
          }
        }
      }
      frame "Run Cmds" {
        n104 = Unbundle By Name(w263) -> ("ADIS16470DevRef.Cmd FIFO"=w273:refnum<k33>)
        n105 = Unbundle By Name(w263) -> ("SPIDevRef"=w262:T18, "ADIS16470DevRef.Status FIFO"=w268:refnum<k33>, "ADIS16470DevRef.Calibration Complete"=w269:refnum<notifier>)
        n106 = RT FIFO Read(0:w273, 1:T24 {"Command"=enum."None", "Data"=0} ("element")) -> (8:w267:refnum<k33>, 9:w266:T24)  [unwired: 2 in, 3 out]
        n107 = Unbundle By Name(w266) -> ("Command"=w265:T30, "Data"=w264:u32)
        n108 = case shown="\"Start Auto SPI\"" w265 {
          tunnel: w263 -> [w275 w280 w288 w293 w307 w316 w361]
          tunnel: w272 -> [w276 w279 w283 w291 w312 w339 w371]
          tunnel: [w276 w279 w282 w290 w312 w322 w359] -> w271
          tunnel: [w275 w278 w288 w294 w306 w315 w361] -> w270
          tunnel: w269 -> [_ _ _ _ w311 _ _]
          tunnel: w268 -> [_ _ _ w298 w309 _ _]
          tunnel: w267 -> [_ _ _ w296 _ w337 w373]
          tunnel: w264 -> [_ _ w284 _ _ _ _]
          tunnel: w263 -> [_ _ _ _ _ w336 w364]
          tunnel: w262 -> [_ _ w281 w289 _ w313 _]
          frame "None", Default {
          }
          frame "Reset" {
            n109 = Bundle By Name(cluster=w280, "Reset"=TRUE ("First Run")) -> (w278:T21)
          }
          frame "Set Calibration Period" {
            w286 = T19 102 items=["Reserved1"=0, "DIAG_STAT"=2, "X_GYRO_LOW"=4, "X_GYRO_OUT"=6, "Y_GYRO_LOW"=8, "Y_GYRO_OUT"=10, "Z_GYRO_LOW"=12, "Z_GYRO_OUT"=14, "X_ACCL_LOW"=16, "X_ACCL_OUT"=18, "Y_ACCL_LOW"=20, "Y_ACCL_OUT"=22, "Z_ACCL_LOW"=24, "Z_ACCL_OUT"=26, "TEMP_OUT"=28, "TIME_STAMP"=30, "Reseved2"=32, "DATA_CNTR"=34, "X_DELTANG_LOW"=36, "X_DELTANG_OUT"=38, "Y_DELTANG_LOW"=40, "Y_DELTANG_OUT"=42, "Z_DELTANG_LOW"=44, "Z_DELTANG_OUT"=46, "X_DELTVEL_LOW"=48, "X_DELTVEL_OUT"=50, "Y_DELTVEL_LOW"=52, "Y_DELTVEL_OUT"=54, "Z_DELTVEL_LOW"=56, "Z_DELTVEL_OUT"=58, "Reserved3"=60, "Reserved4"=62, "XG_BIAS_LOW"=64, "XG_BIAS_HIGH"=66, "YG_BIAS_LOW"=68, "YG_BIAS_OUT"=70, "ZG_BIAS_LOW"=72, "ZG_BIAS_OUT"=74, "XA_BIAS_LOW"=76, "XA_BIAS_HIGH"=78, "YA_BIAS_LOW"=80, "YA_BIAS_OUT"=82, "ZA_BIAS_LOW"=84, "ZA_BIAS_OUT"=86, "Reserved5"=88, "Reserved6"=90, "FILT_CTRL"=92, "Reserved5"=94, "MSC_CTRL"=96, "UP_SCALE"=98, "DEC_RATE"=100, "NULL_CNFG"=102, "GLOB_CMD"=104, "Reserved6"=106, "FIRM_REV"=108, "FIRM_DM"=110, "FIRM_Y"=112, "PROD_ID"=114, "SERIAL_NUM"=116, "USER_SCR1"=118, "USER_SCR2"=120, "USER_SCR3"=122, "FLSHCNT_LOW"=124, "FLSHCNT_HIGH"=126] ("Register")
            w287 = 1792  # Data
            n110 = Or(x=w284, y=w287) -> (x .or. y?=w285:u32)
            n111 = call "ADIS16470 Write Register.vi"("error in (no error)"=w283, "Data"=w285, "Register"=w286, "SPIDevRef in"=w281) -> ("error out"=w282:errorcluster)  [unwired: 6 in, 1 out]
          }
          frame "Recalibrate" {
            w299 = T19 104 items=["Reserved1"=0, "DIAG_STAT"=2, "X_GYRO_LOW"=4, "X_GYRO_OUT"=6, "Y_GYRO_LOW"=8, "Y_GYRO_OUT"=10, "Z_GYRO_LOW"=12, "Z_GYRO_OUT"=14, "X_ACCL_LOW"=16, "X_ACCL_OUT"=18, "Y_ACCL_LOW"=20, "Y_ACCL_OUT"=22, "Z_ACCL_LOW"=24, "Z_ACCL_OUT"=26, "TEMP_OUT"=28, "TIME_STAMP"=30, "Reseved2"=32, "DATA_CNTR"=34, "X_DELTANG_LOW"=36, "X_DELTANG_OUT"=38, "Y_DELTANG_LOW"=40, "Y_DELTANG_OUT"=42, "Z_DELTANG_LOW"=44, "Z_DELTANG_OUT"=46, "X_DELTVEL_LOW"=48, "X_DELTVEL_OUT"=50, "Y_DELTVEL_LOW"=52, "Y_DELTVEL_OUT"=54, "Z_DELTVEL_LOW"=56, "Z_DELTVEL_OUT"=58, "Reserved3"=60, "Reserved4"=62, "XG_BIAS_LOW"=64, "XG_BIAS_HIGH"=66, "YG_BIAS_LOW"=68, "YG_BIAS_OUT"=70, "ZG_BIAS_LOW"=72, "ZG_BIAS_OUT"=74, "XA_BIAS_LOW"=76, "XA_BIAS_HIGH"=78, "YA_BIAS_LOW"=80, "YA_BIAS_OUT"=82, "ZA_BIAS_LOW"=84, "ZA_BIAS_OUT"=86, "Reserved5"=88, "Reserved6"=90, "FILT_CTRL"=92, "Reserved5"=94, "MSC_CTRL"=96, "UP_SCALE"=98, "DEC_RATE"=100, "NULL_CNFG"=102, "GLOB_CMD"=104, "Reserved6"=106, "FIRM_REV"=108, "FIRM_DM"=110, "FIRM_Y"=112, "PROD_ID"=114, "SERIAL_NUM"=116, "USER_SCR1"=118, "USER_SCR2"=120, "USER_SCR3"=122, "FLSHCNT_LOW"=124, "FLSHCNT_HIGH"=126] ("Register")
            w302 = u16 1  # Data
            # "Write Calibration"
            # "GLOB_CMD Timing"
            n112 = RT FIFO Write(0:w298, 1:T22 {"Calibrated?"=FALSE, "IMU Detected?"=TRUE} ("element")) -> ()  [unwired: 3 in, 4 out]
            n113 = RT FIFO Write(0:w296, 1:T24 {"Command"=enum."Start Auto SPI", "Data"=0} ("element")) -> ()  [unwired: 3 in, 4 out]
            n114 = call "ADIS16470 Write Register.vi"("error in (no error)"=w291, "Data"=w302, "Register"=w299, "SPIDevRef in"=w289) -> ("error out"=w301:errorcluster, "SPIDevRef out"=w300:T18)  [unwired: 6 in]
            n115 = flat-sequence {
              tunnel: w301 -> [w304]
              tunnel: [w304] -> w290
              tunnel: w300 -> [_]
              frame #0 {
                n116 = Wait (ms)(milliseconds to wait=u32 50) -> ()  [unwired: 1 out]
              }
            }
            n117 = Bundle By Name(cluster=w293, "Reset"=TRUE) -> (w294:T21)
          }
          frame "Recal Complete" {
            n118 = Send Notification(notification="", notifier=w311) -> ()  [unwired: 1 in, 2 out]
            n119 = RT FIFO Write(0:w309, 1:T22 {"Calibrated?"=TRUE, "IMU Detected?"=TRUE} ("element")) -> ()  [unwired: 3 in, 4 out]
            n120 = Bundle By Name(cluster=w307, "AutoSPI Active?"=TRUE) -> (w306:T21)
          }
          frame "Exit Auto SPI" {
            w332 = T19 114 items=["Reserved1"=0, "DIAG_STAT"=2, "X_GYRO_LOW"=4, "X_GYRO_OUT"=6, "Y_GYRO_LOW"=8, "Y_GYRO_OUT"=10, "Z_GYRO_LOW"=12, "Z_GYRO_OUT"=14, "X_ACCL_LOW"=16, "X_ACCL_OUT"=18, "Y_ACCL_LOW"=20, "Y_ACCL_OUT"=22, "Z_ACCL_LOW"=24, "Z_ACCL_OUT"=26, "TEMP_OUT"=28, "TIME_STAMP"=30, "Reseved2"=32, "DATA_CNTR"=34, "X_DELTANG_LOW"=36, "X_DELTANG_OUT"=38, "Y_DELTANG_LOW"=40, "Y_DELTANG_OUT"=42, "Z_DELTANG_LOW"=44, "Z_DELTANG_OUT"=46, "X_DELTVEL_LOW"=48, "X_DELTVEL_OUT"=50, "Y_DELTVEL_LOW"=52, "Y_DELTVEL_OUT"=54, "Z_DELTVEL_LOW"=56, "Z_DELTVEL_OUT"=58, "Reserved3"=60, "Reserved4"=62, "XG_BIAS_LOW"=64, "XG_BIAS_HIGH"=66, "YG_BIAS_LOW"=68, "YG_BIAS_OUT"=70, "ZG_BIAS_LOW"=72, "ZG_BIAS_OUT"=74, "XA_BIAS_LOW"=76, "XA_BIAS_HIGH"=78, "YA_BIAS_LOW"=80, "YA_BIAS_OUT"=82, "ZA_BIAS_LOW"=84, "ZA_BIAS_OUT"=86, "Reserved5"=88, "Reserved6"=90, "FILT_CTRL"=92, "Reserved5"=94, "MSC_CTRL"=96, "UP_SCALE"=98, "DEC_RATE"=100, "NULL_CNFG"=102, "GLOB_CMD"=104, "Reserved6"=106, "FIRM_REV"=108, "FIRM_DM"=110, "FIRM_Y"=112, "PROD_ID"=114, "SERIAL_NUM"=116, "USER_SCR1"=118, "USER_SCR2"=120, "USER_SCR3"=122, "FLSHCNT_LOW"=124, "FLSHCNT_HIGH"=126] ("ADIS16448 Register")
            n121 = Unbundle By Name(w336) -> ("ADIS16470DevRef.Hardware Config.IMU SPI Bus"=w335:T11, "ADIS16470DevRef.Hardware Config.SPI Clock Rate (Hz)"=w334:dbl, "ADIS16470DevRef.Hardware Config.IMU SPI Mode (3)"=w333:T9)
            n122 = call <vilib>:"WPI_SPIClose.vi"("error in (no error)"=w339, "SPIDevRef"=w313) -> ("error out"=w318:errorcluster)  [unwired: 9 in]
            n123 = call <vilib>:"WPI_DigitalOutputRefNum Registry Get.vi"("error in (no error)"=w318, "refnum name"="470 Status LED") -> ("error out"=w320:errorcluster, "DigitalOutputDevRef"=w319:T25)  [unwired: 8 in]
            n124 = call <vilib>:"WPI_DigitalOutputSetValue.vi"("error in (no error)"=w320, "Value"=TRUE, "DigitalOutputDevRef"=w319) -> ("error out"=w317:errorcluster)  [unwired: 7 in, 1 out]
            n125 = RT FIFO Write(0:w337, 1:T24 {"Command"=enum."Recalibrate", "Data"=0} ("element")) -> ()  [unwired: 3 in, 4 out]
            n126 = call <vilib>:"WPI_SPIOpen.vi"("error in"=w317, "Mode (3)"=w333, "Clock Rate (Hz)"=w334, "SPI Bus"=w335) -> ("error out"=w331:errorcluster, "SPIDevRef"=w324:T18)  [unwired: 6 in]
            n127 = call "ADIS16470 Read Register.vi"("error in (no error)"=w331, "ADIS16470 Register"=w332, "SPIDevRef in"=w324) -> ("error out"=w325:errorcluster, "Register Value"=w323:u16, "SPIDevRef out"=w326:T18)  [unwired: 6 in]
            n128 = Or(x=u16 16982 ("y"), y=u16 16470) -> (x .or. y?=w328:u16)
            n129 = Equal?(x=w328, y=w323) -> (x = y?=w327:bool)
            n130 = case shown="True" w327 {
              tunnel: w326 -> [_ w353]
              tunnel: w325 -> [w342 w352]
              tunnel: [w341 w351] -> w322
              tunnel: w316 -> [w340 w349]
              tunnel: [w340 w348] -> w315
              frame False {
                n131 = case shown="No Error" w342 {
                  selector: w342 -> [w344 w347]
                  tunnel: [w343 w347] -> w341
                  frame No Error {
                    n132 = call <vilib>:"Error Cluster From Error Code.vi"("error in (no error)"=w344, "error message (\"\")"="SPI port did not reset properly" ("error message (\"\")"), "error code (0)"=-8106) -> ("error out"=w343:errorcluster)  [unwired: 6 in]
                  }
                  frame Error {
                  }
                }
              }
              frame True {
                n133 = call <vilib>:"WPI_SPIRefNum Registry Set.vi"("error in (no error)"=w352, "refnum name"="AutoSPI", "SPIDevRef"=w353) -> ("error out"=w351:errorcluster, "SPIDevRef"=w354:T18)  [unwired: 7 in]
                n134 = Bundle By Name(cluster=w349, "SPIDevRef"=w354, "AutoSPI Active?"=FALSE) -> (w348:T21)
              }
            }
          }
          frame "Start Auto SPI" {
            n135 = Unbundle By Name(w364) -> ("Data Ready Source"=w363:T13, "SPIDevRef.SPI Bus"=w358:T11, "ADIS16470DevRef.Hardware Config.Stall Config"=w357:T29, "Data Packet"=w356:T19[])
            n136 = RT FIFO Write(0:w373, 1:T24 {"Command"=enum."Recal Complete", "Data"=0} ("element")) -> ()  [unwired: 3 in, 4 out]
            n137 = call <vilib>:"FPGA_SPI_ConfigureAuto.vi"("SPI Auto Zero Byte Count"=u8 0, "error in"=w371, "SPI Auto TX Byte Array"=w356, "Stall Config"=w357, "SPI Bus"=w358) -> ("error out"=w362:errorcluster)  [unwired: 6 in]
            n138 = call <vilib>:"FPGA_SPI_StartAuto_External.vi"("error in (no error)"=w362, "Falling Edge"=TRUE, "Rising Edge"=FALSE, "Source"=w363) -> ("error out"=w368:errorcluster)  [unwired: 7 in]
            n139 = call <vilib>:"WPI_DigitalOutputRefNum Registry Get.vi"("error in (no error)"=w368, "refnum name"="470 Status LED") -> ("error out"=w367:errorcluster, "DigitalOutputDevRef"=w366:T25)  [unwired: 8 in]
            n140 = call <vilib>:"WPI_DigitalOutputSetValue.vi"("error in (no error)"=w367, "Value"=FALSE, "DigitalOutputDevRef"=w366) -> ("error out"=w359:errorcluster)  [unwired: 7 in, 1 out]
          }
        }
      }
      frame "Close" {
        n141 = call <vilib>:"WPI_DigitalOutputRefNum Registry Get.vi"("refnum name"="470 Status LED") -> ("error out"=w386:errorcluster, "DigitalOutputDevRef"=w385:T25)  [unwired: 9 in]
        n142 = call <vilib>:"WPI_DigitalOutputClose.vi"("error in (no error)"=w386, "DigitalOutputDevRef"=w385) -> ("error out"=w384:errorcluster)  [unwired: 9 in]
        n143 = call <vilib>:"WPI_DigitalOutputRefNum Registry Get.vi"("error in (no error)"=w384, "refnum name"="470 Reset Pin") -> ("error out"=w382:errorcluster, "DigitalOutputDevRef"=w381:T25)  [unwired: 8 in]
        n144 = call <vilib>:"WPI_DigitalOutputClose.vi"("error in (no error)"=w382, "DigitalOutputDevRef"=w381) -> ("error out"=w380:errorcluster)  [unwired: 9 in]
        n145 = call <vilib>:"WPI_SPIRefNum Registry Get.vi"("error in (no error)"=w380, "refnum name"="AutoSPI") -> ("error out"=w378:errorcluster, "SPIDevRef"=w377:T18)  [unwired: 8 in]
        n146 = call <vilib>:"WPI_SPIClose.vi"("error in (no error)"=w378, "SPIDevRef"=w377) -> ()  [unwired: 9 in, 1 out]
      }
    }
  }
